vi "Vision Processing.vi"(8 "error in (no error)":errorcluster) -> ()   [LabVIEW 2018]
uses:
  Vision Support Code/Camera Types.ctl
  Robot Global Data.vi
  <vilib>/Rock Robotics/Network Tables/NT Write Number.vi
  <vilib>/vision/NI_Vision_Development_Module.lvlib
panel:
  in  "Min Component %":dbl=5.0
  out "loop ms":u32
  in  "Display Original":bool
  in  "Display Mask":bool
  out "Instructions:":string="Connect a USB or IP camera to your roboRIO. If using a ring light and retroreflective tape, use Camera Settings outside the loop create a dark image with bright and colorful stripes. If used wihtout a ring light, brighten the images so that stripes are visible.\n\nLED Color can encoded as HSL or related color modes. Calibrate to the same color as the strips being reflected to the camera. Unlike the desktop example, this LED color must be set by hand. You can also put the calibration on the dashboard and send the LED Color to the RT code using Network Tables.\n\nThe Display buttons affects whether images are displayed on the panel. It takes quite a bit of CPU  to compress and transmit the images for display.\n\nAdjust Score Cutoff to make the code more or less picky. If the color is not very unique, you may need to increase the number of particles considered. The diagram uses a Size Limit to ignore colored things that are too small. You may need to adjust it if you are targetting from far away.\n\nResults give you the distance to the target, the center and box in a normalized (-1 to 1) and pixel coordinates.\n\nBe sure to read about setting camera exposure and brightness to help simplify your image and acquire color saturated images.\n\nThere are lots of comments on the diagram to explain the code."
  in  "Color Mode":u16(ring)=3 items=["RGB", "HSL", "HSV", "HSI"]
  in  "Particles":dbl=9.0
  in  "Score Cutoff %":dbl=75.0
  in  "Camera Type":T1=enum."MS HD3000 square"
  out "Result":T2 {"Score" format="%#_3g"; "Pixels"."Rectangle"."Numeric 5" format="%#_3g"; "Pixels"."Rectangle"."Numeric 3" format="%#_3g"; "Pixels"."Rectangle"."Numeric 2" format="%#_3g"; "Pixels"."Rectangle"."Numeric" format="%#_3g"; "Normalized"."Rectangle"."Numeric 5" format="%#_2g"; "Normalized"."Rectangle"."Numeric 3" format="%#_2g"; "Normalized"."Rectangle"."Numeric 2" format="%#_2g"; "Normalized"."Rectangle"."Numeric" format="%#_2g"; "Normalized"."Center"."?" format="%#_3g"; "Normalized"."Center"."?" format="%#_3g"; "Distance (ft)" format="%#_3g"}
  out "Qualified Particles":i32
  out "Mask":T3(plugin-control)
  out "Original Image":T3(plugin-control)
  # "Good target, distance ft"
  # "Bad target"
  # "Score in %"
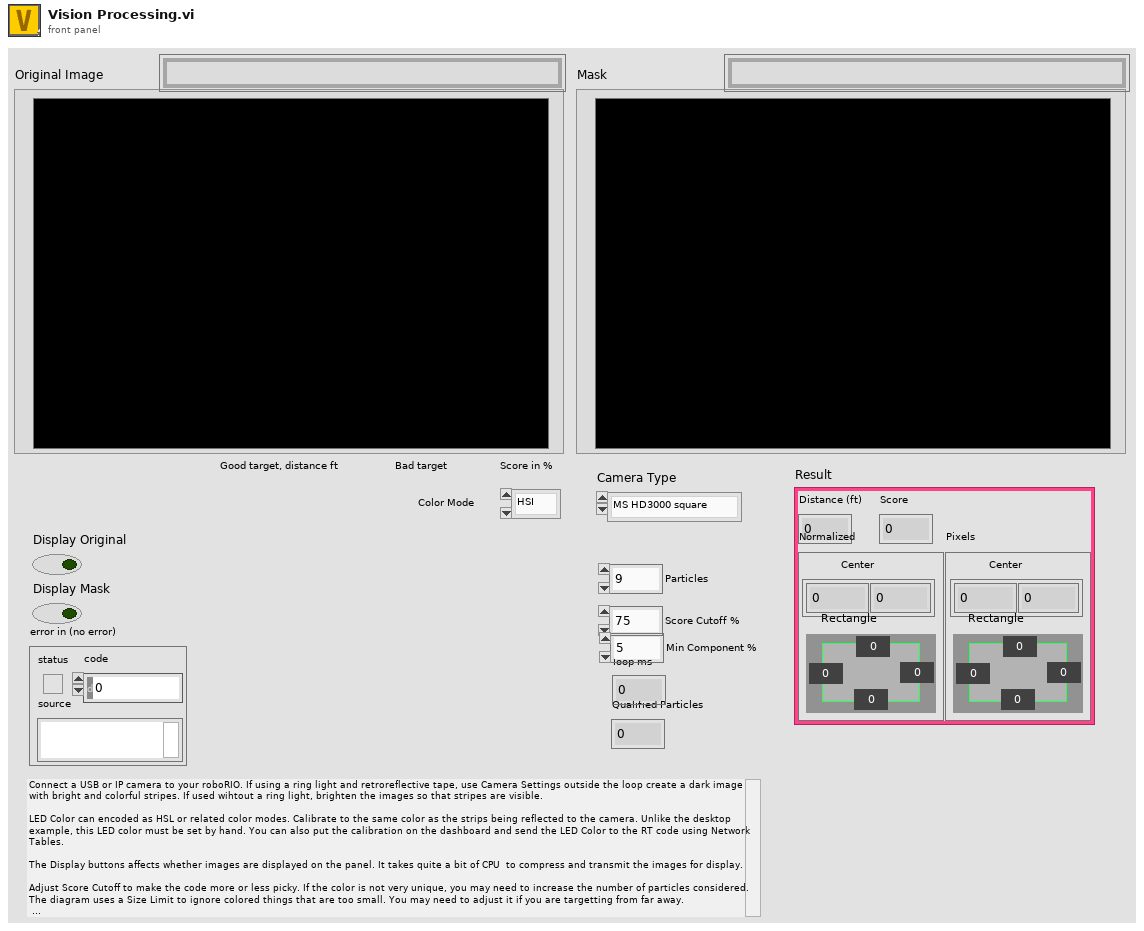
[diagram p1: front panel]
types:
  T1 = typedef "Camera Types.ctl" = enum16{"206", "1011", "1013", "MS HD3000 square", "MS HD3000 640x480"}
  T2 = cluster{"Distance (ft)":dbl, "Score":dbl, "Normalized":cluster{"Center":cluster{dbl, dbl}, "Rectangle":cluster{"Numeric":dbl, "Numeric 2":dbl, "Numeric 3":dbl, "Numeric 5":dbl}}, "Pixels":cluster{"Center":cluster{dbl, dbl}, "Rectangle":cluster{"Numeric":dbl, "Numeric 2":dbl, "Numeric 3":dbl, "Numeric 5":dbl}}}
  T3 = typedef "IMAQ Image.ctl" = refnum<image>
  T4 = typedef "Particle Parameters" = i32
  T5 = typedef "Image Type" = u32
  T6 = typedef "WPI_CameraDevRef.ctl" = cluster{"Camera Address":string, "CameraStatus":errorcluster}
  T7 = cluster{"Hue":cluster{dbl, dbl}, "Sat":cluster{dbl, dbl}, "Val":cluster{dbl, dbl}}
  T8 = typedef "WPI_CameraImageSize.ctl" = enum16{"640x480", "320x240", "160x120", "Custom"}
  T9 = cluster{"Score":dbl, "Rect":cluster{"Left":dbl, "Top":dbl, "Right":dbl, "Bottom":dbl}, "Full Scores":cluster{"Aspect Ratio":dbl, "Top Position":dbl, "Bottom Position":dbl, "Left Gap":dbl, "Width":dbl, "Height Ratio":dbl, "Angle":dbl}}[]
  T10 = cluster{"Score":dbl, "Rect":cluster{"Left":dbl, "Top":dbl, "Right":dbl, "Bottom":dbl}, "Full Scores":cluster{"Aspect Ratio":dbl, "Top Position":dbl, "Bottom Position":dbl, "Left Gap":dbl, "Width":dbl, "Height Ratio":dbl, "Angle":dbl}}
  T11 = cluster{"Left":dbl, "Top":dbl, "Right":dbl, "Bottom":dbl}
  T12 = cluster{"Center":cluster{dbl, dbl}, "Rectangle":cluster{"Numeric":dbl, "Numeric 2":dbl, "Numeric 3":dbl, "Numeric 5":dbl}}
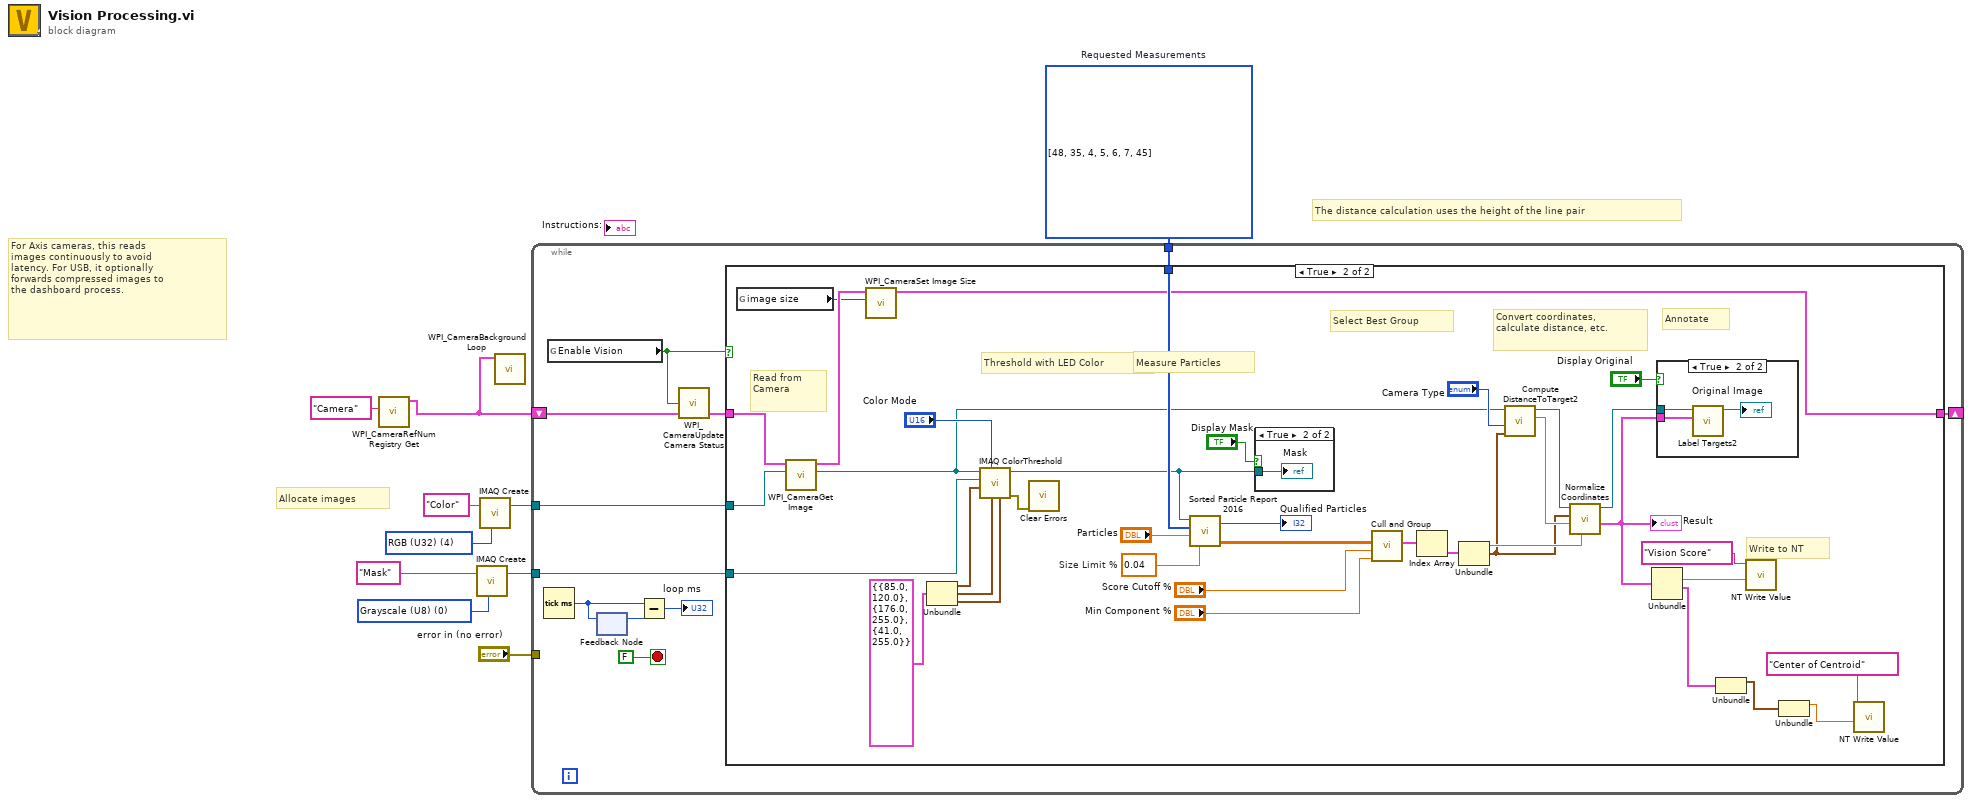
[diagram p0: block diagram]
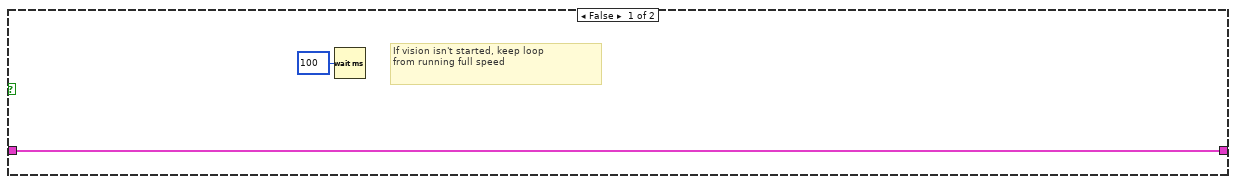
[diagram p2: hidden frame]
diagram:
  w5 = T4[] [48, 35, 4, 5, 6, 7, 45] items=["Center of Mass X", "Center of Mass Y", "First Pixel X", "First Pixel Y", "Bounding Rect Left", "Bounding Rect Top", "Bounding Rect Right", "Bounding Rect Bottom", "Max Feret Diameter Start X", "Max Feret Diameter Start Y", "Max Feret Diameter End X", "Max Feret Diameter End Y", "Max Horiz. Segment Length Left", "Max Horiz. Segment Length Right", "Max Horiz. Segment Length Row", "-", "Bounding Rect Width", "Bounding Rect Height", "Bounding Rect Diagonal", "Perimeter", "Convex Hull Perimeter", "Holes' Perimeter", "Max Feret Diameter", "Equivalent Ellipse Major Axis", "Equivalent Ellipse Minor Axis", "Equivalent Ellipse Minor Axis (Feret)", "Equivalent Rect Long Side", "Equivalent Rect Short Side", "Equivalent Rect Diagonal", "Equivalent Rect Short Side (Feret)", "Average Horiz. Segment Length", "Average Vert. Segment Length", "Hydraulic Radius", "Waddel Disk Diameter", "-", "Area", "Holes' Area", "Particle & Holes' Area", "Convex Hull Area", "Image Area", "-", "Number of Holes", "Number of Horiz. Segments", "Number of Vert. Segments", "-", "Orientation", "Max Feret Diameter Orientation", "-", "% Area/Image Area", "% Area/(Particle & Holes' Area)", "Ratio of Equivalent Ellipse Axes", "Ratio of Equivalent Rect Sides", "-", "Elongation Factor", "Compactness Factor", "Heywood Circularity Factor", "Type Factor", "-", "Sum X", "Sum Y", "Sum XX", "Sum XY", "Sum YY", "Sum XXX", "Sum XXY", "Sum XYY", "Sum YYY", "-", "Moment of Inertia XX", "Moment of Inertia XY", "Moment of Inertia YY", "Moment of Inertia XXX", "Moment of Inertia XXY", "Moment of Inertia XYY", "Moment of Inertia YYY", "Norm. Moment of Inertia XX", "Norm. Moment of Inertia XY", "Norm. Moment of Inertia YY", "Norm. Moment of Inertia XXX", "Norm. Moment of Inertia XXY", "Norm. Moment of Inertia XYY", "Norm. Moment of Inertia YYY", "Hu Moment 1", "Hu Moment 2", "Hu Moment 3", "Hu Moment 4", "Hu Moment 5", "Hu Moment 6", "Hu Moment 7"]  # Requested Measurements
  w8 = T5 0 items=["Grayscale (U8)", "Grayscale (I16)", "Grayscale (SGL)", "Complex (CSG)", "RGB (U32)", "HSL (U32)", "RGB (U64)", "Grayscale (U16)"] ("Image Type")
  w9 = T5 4 items=["Grayscale (U8)", "Grayscale (I16)", "Grayscale (SGL)", "Complex (CSG)", "RGB (U32)", "HSL (U32)", "RGB (U64)", "Grayscale (U16)"] ("Image Type")
  # "For Axis cameras, this reads\nimages continuously to avoid\nlatency. For USB, it optionally\nforwards compressed images to\nthe dashboard process."
  # "The distance calculation uses the height of the line pair"
  # "Allocate images"
  n1 = call <vilib>:"WPI_CameraRefNum Registry Get.vi"("refnum name"="Camera") -> ("CameraDevRef"=w2:T6)  [unwired: 9 in, 1 out]
  n2 = call "IMAQ Create"("Image Name"="Mask", "Image Type"=w8) -> ("New Image"=w6:T3)  [unwired: 2 in, 2 out]
  n3 = call "IMAQ Create"("Image Name"="Color", "Image Type"=w9) -> ("New Image"=w4:T3)  [unwired: 2 in, 2 out]
  n4 = call <vilib>:"WPI_CameraBackground Loop.vi"("CameraDevRef"=w2) -> ()  [unwired: 11 in]
  n5 = while {
    tunnel: w4 -> [w18]
    tunnel: w6 -> [w20]
    tunnel: w5 -> [w19]
    shift-right: [w17] -> _
    shift-left: w2 -> [w16]
    tunnel: "error in (no error)" -> [_]
    stop <- FALSE stop-if-true
    n6 = Tick Count (ms)() -> (millisecond timer value=w12:u32)
    n7 = global read "Robot Global Data.vi" "Enable Vision"() -> (w14:bool)
    n8 = feedback-in #1(w12) -> ()
    n9 = feedback #1() -> (w13:u32)  [unwired: 1 in]
    n10 = Subtract(x=w12, y=w13) -> (x-y=→"loop ms":u32)
    n11 = call <vilib>:"WPI_CameraUpdate Camera Status.vi"("CameraDevRef In"=w16, "Enable Vision"=w14) -> ("CameraDevRef Out"=w15:T6)  [unwired: 3 in]
    n12 = case shown="True" w14 {
      tunnel: w20 -> [_ w61]
      tunnel: w19 -> [_ w57]
      tunnel: w15 -> [w23 w44]
      tunnel: w18 -> [_ w43]
      tunnel: [w23 w38] -> w17
      frame False {
        # "If vision isn't started, keep loop\nfrom running full speed"
        n13 = Wait (ms)(milliseconds to wait=u32 100) -> ()  [unwired: 1 out]
      }
      frame True {
        w55 = 0.04  # Size Limit %
        # "Write to NT"
        # "Read from\nCamera"
        # "Measure Particles"
        # "Convert coordinates,\ncalculate distance, etc."
        # "Annotate"
        # "Select Best Group"
        # "Threshold with LED Color"
        n14 = global read "Robot Global Data.vi" "image size"() -> (w37:T8)
        n15 = call <vilib>:"WPI_CameraGet Image.vi"("Image"=w43, "CameraDevRef"=w44) -> ("Image Out"=w42:T3, "CameraDevRef Out"=w39:T6)  [unwired: 7 in, 1 out]
        n16 = call <vilib>:"WPI_CameraSet Image Size.vi"("Image Size"=w37, "CameraDevRef"=w39) -> ("CameraDevRef Out"=w38:T6)  [unwired: 2 in, 7 out]
        n17 = Unbundle(T7 {"Hue"={85.0, 120.0}, "Sat"={176.0, 255.0}, "Val"={41.0, 255.0}} ("cluster")) -> ("Hue"=w60:cluster{dbl, dbl}, "Sat"=w59:cluster{dbl, dbl}, "Val"=w58:cluster{dbl, dbl})
        n18 = call "IMAQ ColorThreshold"("Blue or Luma or Val or Inten Range"=w58, "Green or Sat Range"=w59, "Color Mode"="Color Mode", "Red or Hue Range"=w60, "Image Dst"=w61, "Image Src"=w42) -> ("error out"=w54:errorcluster, "Image Dst Out"=w51:T3)  [unwired: 4 in]
        n19 = call <vilib>:"Clear Errors.vi"("error in (no error)"=w54) -> ()  [unwired: 5 in, 2 out]
        n20 = call "Sorted Particle Report 2016.vi"("Min Area Size %"=w55, "Particle Count Limit"="Particles", "Pixel Measurements"=w57, "Image in"=w51) -> ("Sorted Data"=w53:dbl[][], "Particles"=→"Qualified Particles":i32)
        n21 = case shown="True" "Display Mask" {
          tunnel: w51 -> [_ w65]
          frame False {
          }
          frame True {
            "Mask" <- w65
          }
        }
        n22 = call "Cull and Group.vi"("Min Compnt %"="Min Component %", "Score Cutoff %"="Score Cutoff %", "Sorted Data"=w53) -> ("Best Targets above cutoff"=w33:T9)  [unwired: 8 in]
        n23 = Index Array(array=w33) -> (element=w32:T10)  [unwired: 1 in]
        n24 = Unbundle(w32) -> ("Score"=w31:dbl, "Rect"=w30:T11)  [unwired: 1 out]
        n25 = call "Compute DistanceToTarget2.vi"("Rect"=w30, "Camera Type"="Camera Type", "Image Src"=w42) -> ("Distance (ft)"=w49:dbl, "Image Dst Out"=w48:T3)  [unwired: 7 in]
        n26 = call "Normalize Coordinates.vi"("Score"=w31, "Distance"=w49, "Bounding box"=w30, "Image in"=w48) -> ("Results"=w36:T2, "Image out"=w47:T3)  [unwired: 6 in]
        "Result" <- w36
        n27 = Unbundle(w36) -> ("Score"=w35:dbl, "Normalized"=w28:T12)  [unwired: 2 out]
        n28 = case shown="True" "Display Original" {
          tunnel: w47 -> [_ w63]
          tunnel: w36 -> [_ w62]
          frame False {
          }
          frame True {
            n29 = call "Label Targets2.vi"("Results"=w62, "Image in"=w63) -> ("Image out"=→"Original Image":T3)  [unwired: 9 in]
          }
        }
        n30 = Unbundle(w28) -> ("Center"=w27:cluster{dbl, dbl})  [unwired: 1 out]
        n31 = call-poly <vilib>:"NT Write Value.vi"("Numeric"=w35, "Name"="Vision Score") -> ()  [unwired: 9 in, 1 out]
        n32 = Unbundle(w27) -> (w26:dbl)  [unwired: 1 out]
        n33 = call-poly <vilib>:"NT Write Value.vi"("Numeric"=w26, "Name"="Center of Centroid") -> ()  [unwired: 9 in, 1 out]
      }
    }
  }
